vi "Prepare Channel Names.vi"(10 "#Outputs":i32, 11 "#Inputs":i32) -> (3 "Channel Names":string[](array[string]))   [LabVIEW 2015, in "Teaching File.lvlib"]
doc: "Prepare a list of names for IO channels, based on the numbers of IO."
uses:
  Teaching File.lvlib
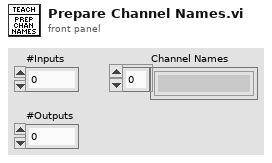
[diagram p1: front panel]
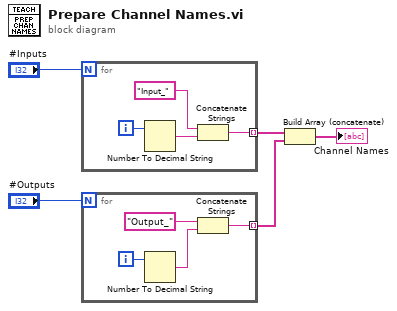
[diagram p0: block diagram]
diagram:
  n1 = for {
    N: "#Inputs" -> [_]
    tunnel: [w6] -> w1 mode=indexing
    i -> [w8]
    n2 = Number To Decimal String(number=w8) -> (decimal integer string=w9:string)  [unwired: 1 in]
    n3 = Concatenate Strings("Input_" ("group name in"), w9) -> (w6:string)
  }
  n4 = for {
    N: "#Outputs" -> [_]
    tunnel: [w10] -> w2 mode=indexing
    i -> [w12]
    n5 = Number To Decimal String(number=w12) -> (decimal integer string=w13:string)  [unwired: 1 in]
    n6 = Concatenate Strings("Output_" ("group name in"), w13) -> (w10:string)
  }
  n7 = Build Array (concatenate)(w1, w2) -> (→"Channel Names":string[])
